vi "File_checker_and_finder.vi"(2 "Promp if not found":string, 3 "Filename In":path) -> (0 "cancelled":bool, 1 "Filename Out":path)   [LabVIEW 2021]
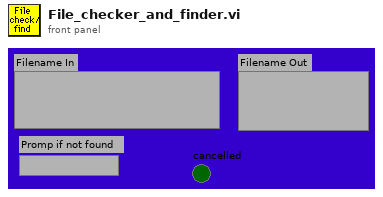
[diagram p1: front panel]
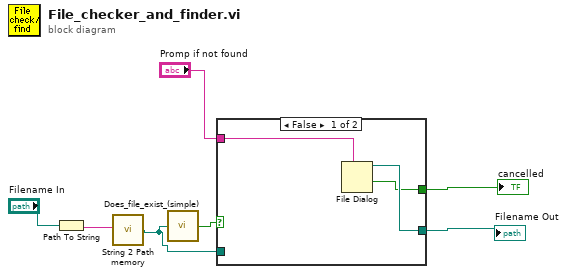
[diagram p0: block diagram]
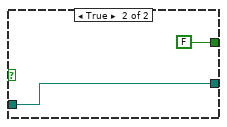
[diagram p2: hidden frame]
diagram:
  n1 = Path To String(path="Filename In") -> (string=w2:string)
  n2 = call "String 2 Path memory.vi"("Input String"=w2) -> ("path"=w1:path)  [unwired: 1 in]
  n3 = call "Does_file_exist_(simple).vi"("Pathname"=w1) -> ("exists?"=w4:bool)
  n4 = case shown="False" w4 {
    tunnel: "Promp if not found" -> [w10 _]
    tunnel: [w9 w12] -> w7
    tunnel: [w8 FALSE ("cancelled")] -> w5
    tunnel: w1 -> [_ w12]
    frame False {
      n5 = File Dialog(7:w10) -> (1:w8:bool, 3:w9:path)  [unwired: 1 in, 7 out]
    }
    frame True {
    }
  }
  "Filename Out" <- w7
  "cancelled" <- w5
